vi "Set Scan Rate.vi"(5 "System Definition Dir":path, 6 "IP address":string, 7 "Details Ref":refnum<vi>, 8 "error in (no error)":errorcluster, 10 "WebDAV session in":T1, 11 "Device Item Ref in":T2 format="%.0x") -> (0 "error out":errorcluster, 2 "WebDAV session out":T1, 3 "Device Item Ref out":T2 format="%.0x")   [LabVIEW 2024, in "SEECD System Explorer.lvlib"]
uses:
  SEECD System Explorer.lvlib
  <vilib>/NI VeriStand/Custom Device API/Custom Device Item Ref.ctl
  <vilib>/WebDAVClient/Advanced/SessionHandle.ctl
  Shared/Globals/Property Strings.vi
  <vilib>/NI VeriStand/Custom Device API/Custom Device API.lvlib
  Shared/SEECD Shared.lvlib
  <vilib>/WebDAVClient/NI_WebDAV.lvlib
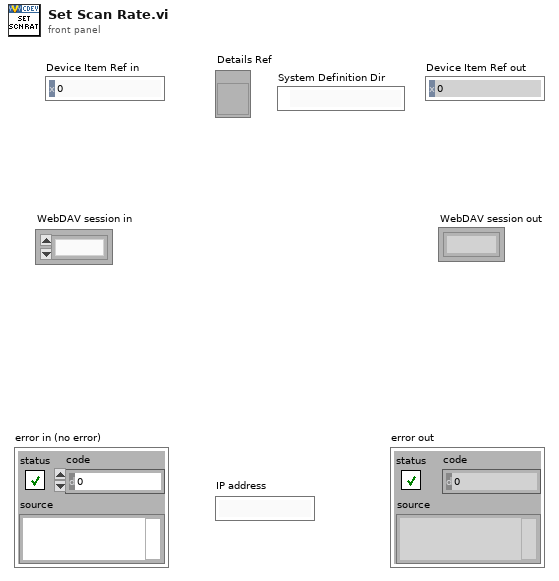
[diagram p1: front panel]
types:
  T1 = typedef "NI_WebDAV.lvlib/SessionHandle.ctl" = refnum<k1>
  T2 = typedef "Custom Device API.lvlib/Custom Device Item Ref.ctl" = u64
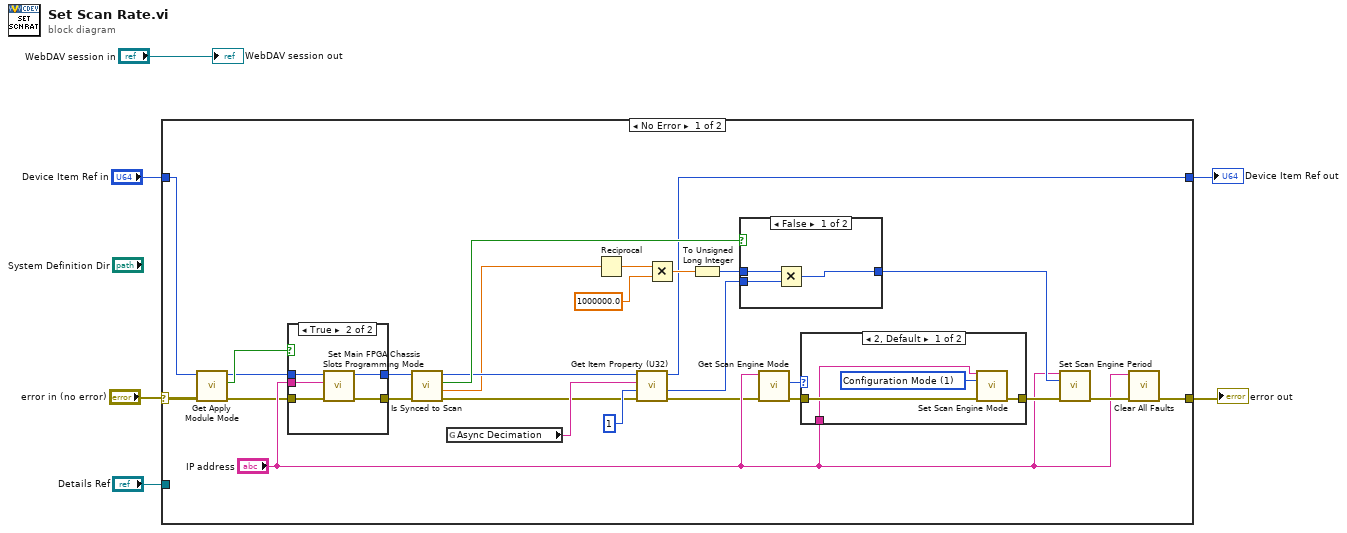
[diagram p0: block diagram]
diagram:
  n1 = case shown="No Error" "error in (no error)" {
    selector: "error in (no error)" -> [w12 w51]
    tunnel: [w16 w51] -> w1
    tunnel: "Device Item Ref in" -> [w11 w50]
    tunnel: [w7 w50] -> w2
    tunnel: "Details Ref" -> [_ _]
    frame No Error {
      n2 = call "Get Apply Module Mode.vi"("error in (no error)"=w12, "Device Item Ref in"=w11) -> ("error out"=w10:errorcluster, "Apply Module Mode"=w9:bool, "Device Item Ref out"=w8:T2)  [unwired: 7 in]
      n3 = case shown="True" w9 {
        tunnel: w8 -> [w44 w49]
        tunnel: "IP address" -> [_ w48]
        tunnel: [w43 w47] -> w14
        tunnel: [w44 w46] -> w13
        tunnel: w10 -> [w43 w45]
        frame False {
        }
        frame True {
          n4 = call "Set Main FPGA Chassis Slots Programming Mode.vi"("error in (no error)"=w45, "serverName in"=w48, "Item Ref in"=w49) -> ("error out"=w47:errorcluster, "Item Ref out"=w46:T2)  [unwired: 6 in, 1 out]
        }
      }
      n5 = call "Is Synced to Scan.vi"("error in"=w14, "Item Ref in"=w13) -> ("error out"=w20:errorcluster, "Engine Rate"=w18:dbl, "Sync to Scan?"=w25:bool, "Item Ref out"=w19:T2)  [unwired: 6 in]
      n6 = global read "Property Strings.vi" "Async Decimation"() -> (w29:string)
      n7 = Reciprocal(x=w18) -> (1/x=w22:dbl)
      n8 = call <vilib>:"Get Item Property (U32).vi"("error in (no error)"=w20, "Default Value"=u32 1, "Property Name"=w29, "Item Ref in"=w19) -> ("error out"=w15:errorcluster, "Value"=w23:u32, "Item Ref out"=w7:T2)  [unwired: 4 in, 1 out]
      n9 = Multiply(x=w22, y=1000000.0) -> (x*y=w28:dbl)
      n10 = To Unsigned Long Integer(number=w28) -> (unsigned 32bit integer=w21:u32)
      n11 = case shown="False" w25 {
        tunnel: w21 -> [w41 w42]
        tunnel: w23 -> [w40 _]
        tunnel: [w39 w42] -> w24
        frame False {
          n12 = Multiply(x=w41, y=w40) -> (x*y=w39:u32)
        }
        frame True {
        }
      }
      n13 = call <vilib>:"Get Scan Engine Mode.vi"("error in (no error)"=w15, "target address (localhost)"="IP address") -> ("error out"=w31:errorcluster, "mode"=w32:i32)  [unwired: 8 in]
      n14 = case shown="2, Default" w32 {
        tunnel: w31 -> [w36 w38]
        tunnel: [w35 w38] -> w33
        tunnel: "IP address" -> [w34 _]
        frame 2, Default {
          w37 = 1 items=["Configuration Mode"=1, "Active Mode"=2] ("mode (Active Mode)")
          n15 = call <vilib>:"Set Scan Engine Mode.vi"("target address (localhost)"=w34, "mode (Active Mode)"=w37, "error in (no error)"=w36) -> ("error out"=w35:errorcluster)  [unwired: 12 in]
        }
        frame 1 {
        }
      }
      n16 = call <vilib>:"Set Scan Engine Period.vi"("target address (localhost)"="IP address", "scan period (uSec)"=w24, "error in (no error)"=w33) -> ("error out"=w26:errorcluster)  [unwired: 12 in]
      n17 = call <vilib>:"Clear All Faults.vi"("error in (no error)"=w26, "target address (localhost)"="IP address") -> ("error out"=w16:errorcluster)  [unwired: 9 in]
    }
    frame Error {
    }
  }
  "error out" <- w1
  "Device Item Ref out" <- w2
  "WebDAV session out" <- "WebDAV session in"
